vi "Type.vi"(11 "TimestampPanel in":refnum<class "TimestampPanel.lvclass">) -> (2 "Type":refnum<class "Type.lvclass">)   [LabVIEW 2020, in "Conditum-Tools.lvlib" / "TimestampPanel.lvclass"]
uses:
  TimestampPanel.lvclass
  Conditum/Columns/Type/Type.lvclass
  TimestampPanel.lvclass/TimestampPanel.ctl
  Conditum/Columns/Timestamp/Timestamp.lvclass
  C:/dev/lv20CE/lv-conditum/Conditum/Columns/Type/Type.lvclass
  C:/dev/lv20CE/lv-conditum/Conditum/Columns/Timestamp/Timestamp.lvclass
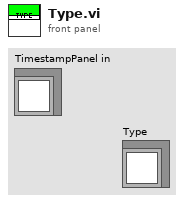
[diagram p1: front panel]
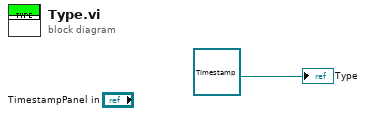
[diagram p0: block diagram]
diagram:
  "Type" <- refnum<class "Timestamp.lvclass"> refnum ("Conditum:Columns:Timestamp.lvclass")
